vi "niScope Set PFI.vi"(8 "error in":errorcluster, 10 "PFI state":enum16{"None", "PFI 0", "PFI 1"}(ring), 11 "instrument handle":refnum<k15>) -> (0 "error out":errorcluster)   [LabVIEW 2020, in "niScope Virtual Digitizer.lvlib"]
doc: "This VI sets reference clock output to the selected PFI line (or none). It is used mainly to control a multiplexer (after rectifying the signal)."
uses:
  niScope Virtual Digitizer.lvlib
  <instrlib>/niScope/Controls/niScope exportable signals.ctl
  <instrlib>/niScope/Controls/niScope export destinations.ctl
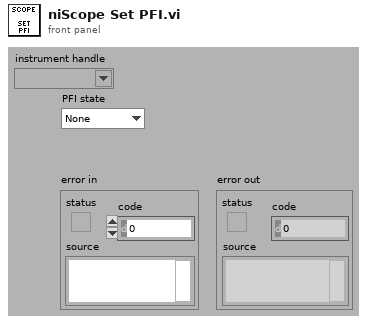
[diagram p1: front panel]
types:
  T1 = typedef "niScope export destinations.ctl" = string
  T2 = typedef "niScope exportable signals.ctl" = u16
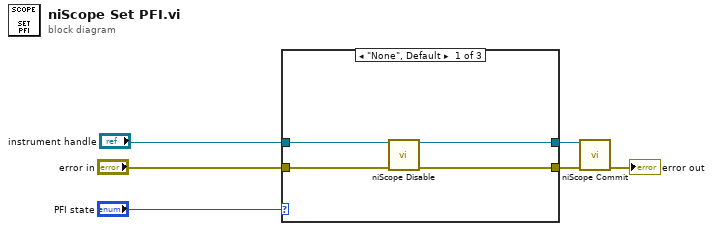
[diagram p0: block diagram]
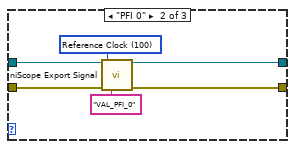
[diagram p2: hidden frame]
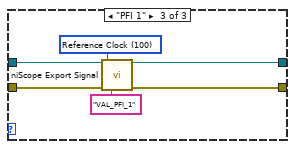
[diagram p3: hidden frame]
diagram:
  n1 = case shown="\"None\", Default" "PFI state" {
    tunnel: [w7 w12 w17] -> w3
    tunnel: "instrument handle" -> [w9 w16 w19]
    tunnel: "error in" -> [w10 w15 w22]
    tunnel: [w8 w11 w18] -> w1
    frame "None", Default {
      n2 = call <instrlib>:"niScope Disable.vi"("instrument handle"=w9, "error in"=w10) -> ("instrument handle out"=w8:refnum<k15>, "error out"=w7:errorcluster)  [unwired: 12 in]
    }
    frame "PFI 0" {
      w14 = T2 100 items=["None"=0, "Start Trigger"=2, "Advance Trigger"=5, "Reference Trigger"=1, "End of Record Event"=4, "End of Acquisition Event"=3, "Ready for Start Event"=7, "Ready for Advance Event"=6, "Ready for Reference Event"=10, "Reference Clock"=100, "Sample Clock"=101, "5 Volt Power"=13] ("signal")
      n3 = call <instrlib>:"niScope Export Signal.vi"("instrument handle"=w16, "signal"=w14, "output terminal"=T1 "VAL_PFI_0", "error in"=w15) -> ("instrument handle out"=w11:refnum<k15>, "error out"=w12:errorcluster)  [unwired: 10 in]
    }
    frame "PFI 1" {
      w21 = T2 100 items=["None"=0, "Start Trigger"=2, "Advance Trigger"=5, "Reference Trigger"=1, "End of Record Event"=4, "End of Acquisition Event"=3, "Ready for Start Event"=7, "Ready for Advance Event"=6, "Ready for Reference Event"=10, "Reference Clock"=100, "Sample Clock"=101, "5 Volt Power"=13] ("signal")
      n4 = call <instrlib>:"niScope Export Signal.vi"("instrument handle"=w19, "signal"=w21, "output terminal"=T1 "VAL_PFI_1", "error in"=w22) -> ("instrument handle out"=w18:refnum<k15>, "error out"=w17:errorcluster)  [unwired: 10 in]
    }
  }
  n5 = call <instrlib>:"niScope Commit.vi"("instrument handle"=w1, "error in"=w3) -> ("error out"=→"error out":errorcluster)  [unwired: 12 in, 1 out]
